vi "Begin.vi"(8 "error in":errorcluster) -> (0 "error out":errorcluster)   [LabVIEW 2020]
doc: "Called before other user functions, this VI is expected to open initial I/O refnums, load in file data, and do all program initialization. Notice that the <B>error out</B> terminal is simply used for data flow. Wiring it to other structures or subVIs ensures that this VI runs first."
uses:
  <vilib>/Rock Robotics/WPI/DriverStation/WPI_DriverStationRobotMode2.ctl
  <vilib>/Rock Robotics/WPI/Joystick/WPI_JoystickDeviceEnum.ctl
  <vilib>/Rock Robotics/WPI/Compressor/WPI_CompressorFeedbackMode.ctl
  Robot Global Data.vi
  <vilib>/Rock Robotics/WPI/Utilities/WPI_GetSetVariantRefNum.vi
  Globals/Calibration_And_Constant_Globals.vi
  Globals/FilePath_Globals.vi
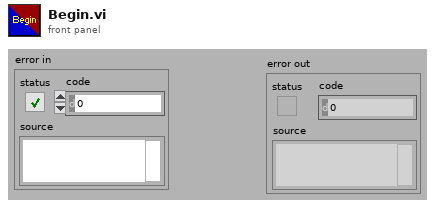
[diagram p1: front panel]
types:
  T1 = typedef "WPI_JoystickDeviceEnum.ctl" = enum16{"USB 0", "USB 1", "USB 2", "USB 3", "USB 4", "USB 5"}
  T2 = typedef "WPI_DriverStationRobotMode2.ctl" = enum16{"Autonomous Disabled", "Autonomous Enabled", "Teleop Disabled", "Teleop Enabled", "Disconnected", "Finish", "Test Disabled", "Test Enabled", "Emergency Stopped"}
  T3 = typedef "WPI_CompressorFeedbackMode.ctl" = enum16{"Analog Only", "Digital Only", "Hybrid"}
  T4 = cluster{"Feedback Sensor":T3, "Max Pressure (PSI)":dbl, "Min Pressure (PSI)":dbl}
  T5 = typedef "WPI_CompressorDevRef.ctl" = cluster{"DevStatus":errorcluster, "Pneumatics Control Module":u8}
  T6 = typedef "WPI_JoystickDevRef.ctl" = cluster{"Device":T1}
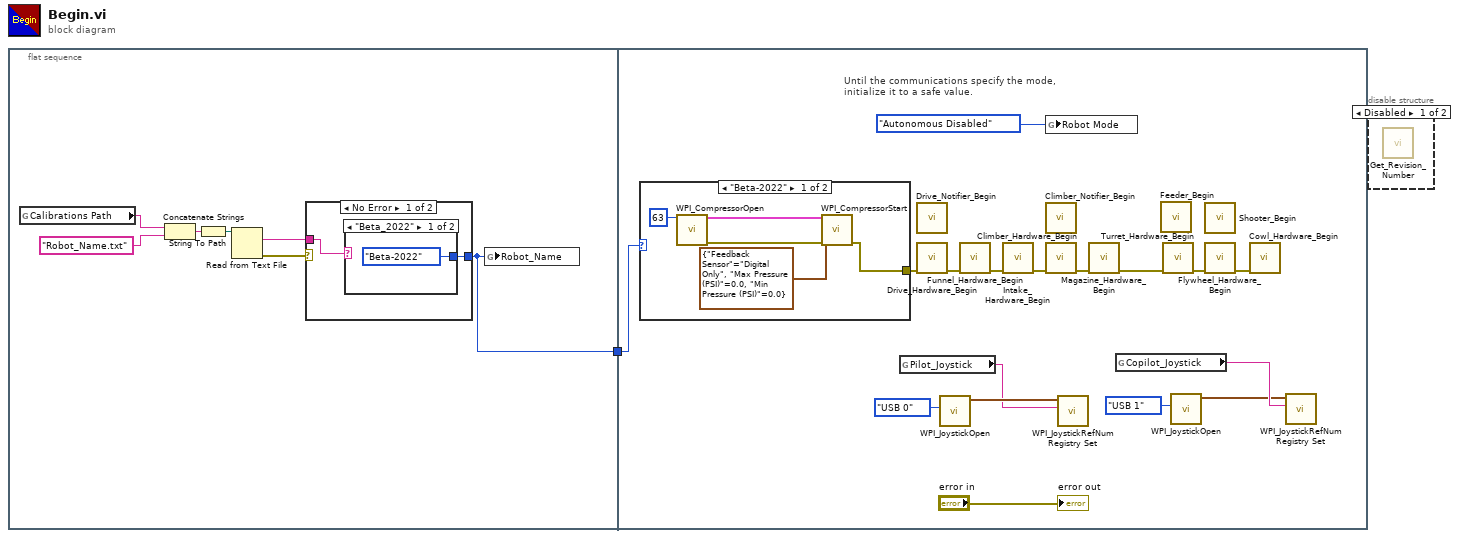
[diagram p0: block diagram]
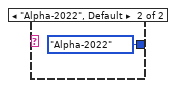
[diagram p2: hidden frame]
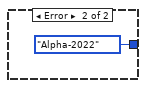
[diagram p3: hidden frame]
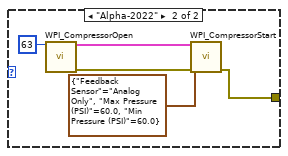
[diagram p4: hidden frame]
diagram:
  n1 = flat-sequence {
    tunnel: [w2] -> w1
    tunnel: w1 -> [w15]
    frame #0 {
      n2 = global read "FilePath_Globals.vi" "Calibrations Path"() -> (w8:string)
      n3 = Concatenate Strings(w8, "Robot_Name.txt" ("string")) -> (w6:string)
      n4 = String To Path(string=w6) -> (path=w5:path)
      n5 = Read from Text File(file (use dialog)=w5) -> (text=w3:string, error out=w4:errorcluster)  [unwired: 3 in, 2 out]
      n6 = case shown="No Error" w4 {
        tunnel: w3 -> [w10 _]
        tunnel: [w9 enum16{"Alpha-2022", "Beta-2022"}."Alpha-2022" ("Robot_Name")] -> w2
        frame No Error {
          n7 = case shown="\"Beta_2022\"" w10 {
            tunnel: [enum16{"Alpha-2022", "Beta-2022"}."Beta-2022" ("Robot_Name") enum16{"Alpha-2022", "Beta-2022"}."Alpha-2022" ("Robot_Name")] -> w9
            frame "Beta_2022" {
            }
            frame "Alpha-2022", Default {
            }
          }
        }
        frame Error {
        }
      }
      n8 = global write "Calibration_And_Constant_Globals.vi" "Robot_Name"(w2) -> ()
    }
    frame #1 {
      # "Until the communications specify the mode,\ninitialize it to a safe value."
      n9 = case shown="\"Beta-2022\"" w15 {
        tunnel: [w31 w36] -> w14
        frame "Beta-2022" {
          n10 = call <vilib>:"WPI_CompressorOpen.vi"("Pneumatics device (def)"=u8 63) -> ("CompressorDevRef"=w34:T5, "error out"=w35:errorcluster)  [unwired: 13 in]
          n11 = call <vilib>:"WPI_CompressorStart.vi"("error in (no error)"=w35, "Feedback Configuration"=T4 {"Feedback Sensor"=enum."Digital Only", "Max Pressure (PSI)"=0.0, "Min Pressure (PSI)"=0.0}, "CompressorDevRef"=w34) -> ("error out"=w31:errorcluster)  [unwired: 7 in, 1 out]
        }
        frame "Alpha-2022" {
          n12 = call <vilib>:"WPI_CompressorOpen.vi"("Pneumatics device (def)"=u8 63) -> ("CompressorDevRef"=w39:T5, "error out"=w40:errorcluster)  [unwired: 13 in]
          n13 = call <vilib>:"WPI_CompressorStart.vi"("error in (no error)"=w40, "Feedback Configuration"=T4 {"Feedback Sensor"=enum."Analog Only", "Max Pressure (PSI)"=60.0, "Min Pressure (PSI)"=60.0}, "CompressorDevRef"=w39) -> ("error out"=w36:errorcluster)  [unwired: 7 in, 1 out]
        }
      }
      n14 = global read "Calibration_And_Constant_Globals.vi" "Pilot_Joystick"() -> (w27:string)
      n15 = call "Drive_Notifier_Begin.vi"() -> ()  [unwired: 12 in]
      n16 = call "Drive_Hardware_Begin.vi"("error in"=w14) -> ("error out"=w18:errorcluster)  [unwired: 10 in]
      n17 = call <vilib>:"WPI_JoystickOpen.vi"("JoystickDevice"=WPI_JoystickDeviceEnum."USB 0") -> ("JoystickDevRef"=w30:T6)  [unwired: 10 in]
      n18 = call "Funnel_Hardware_Begin.vi"("error in"=w18) -> ("error out"=w22:errorcluster)  [unwired: 10 in]
      n19 = call "Intake_Hardware_Begin.vi"("error in"=w22) -> ("error out"=w21:errorcluster)  [unwired: 10 in]
      n20 = global write "Robot Global Data.vi" "Robot Mode"(WPI_DriverStationRobotMode2."Autonomous Disabled" ("Robot Mode")) -> ()
      n21 = call "Climber_Notifier_Begin.vi"() -> ()  [unwired: 12 in]
      n22 = call "Climber_Hardware_Begin.vi"("error in"=w21) -> ("error out"=w20:errorcluster)  [unwired: 10 in]
      n23 = call <vilib>:"WPI_JoystickRefNum Registry Set.vi"("refnum name"=w27, "JoystickDevRef"=w30) -> ()  [unwired: 8 in, 2 out]
      n24 = call "Magazine_Hardware_Begin.vi"("error in"=w20) -> ("error out"=w19:errorcluster)  [unwired: 10 in]
      n25 = global read "Calibration_And_Constant_Globals.vi" "Copilot_Joystick"() -> (w26:string)
      n26 = call "Feeder_Begin.vi"() -> ()  [unwired: 12 in]
      n27 = call "Turret_Hardware_Begin.vi"("error in"=w19) -> ("error out"=w17:errorcluster)  [unwired: 10 in]
      n28 = call <vilib>:"WPI_JoystickOpen.vi"("JoystickDevice"=WPI_JoystickDeviceEnum."USB 1") -> ("JoystickDevRef"=w24:T6)  [unwired: 10 in]
      n29 = call "Shooter_Begin.vi"() -> ()  [unwired: 12 in]
      n30 = call "Flywheel_Hardware_Begin.vi"("error in"=w17) -> ("error out"=w16:errorcluster)  [unwired: 10 in]
      n31 = call "Cowl_Hardware_Begin.vi"("error in"=w16) -> ()  [unwired: 10 in, 1 out]
      n32 = call <vilib>:"WPI_JoystickRefNum Registry Set.vi"("refnum name"=w26, "JoystickDevRef"=w24) -> ()  [unwired: 8 in, 2 out]
      "error out" <- "error in"
    }
  }
  n33 = disable-structure shown="Disabled" {
    frame Disabled {
      n34 = call "Get_Revision_Number.vi"() -> ()  [unwired: 1 in, 1 out]
    }
    frame Enabled {
    }
  }
